vi "Teleop.vi"(10 "Match Info":T1={"Autonomous Elapsed Seconds"=0.0, "TeleOp Elapsed Seconds"=0.0, "Disabled Elapsed Seconds"=0.0, "Visited Autonomous"=FALSE, "Visited TeleOp"=FALSE, "Visited Disabled"=FALSE, "Autonomous Settings"={"Autonomous Style"=enum."Independent", "VI Refnum"=refnum}}, 11 "Call Context":T2) -> ()   [LabVIEW 2018]
doc: "This VI is called for each enabled TeleOp packet received from the DS. It is typically used to read from joysticks and other inputs and update I/O or setpoints for timed control loops. It should complete and return within 20 milliseconds or risk missing DS packets."
uses:
  <vilib>/Rock Robotics/WPI/DriverStation/WPI_DriverStationDerivedRobotMode.ctl
  <vilib>/Rock Robotics/WPI/DriverStation/WPI_DriverStationMatch Info.ctl
  <vilib>/Rock Robotics/WPI/Solenoid/WPI_SolenoidValue.ctl
  Framework/Robot Global Data.vi
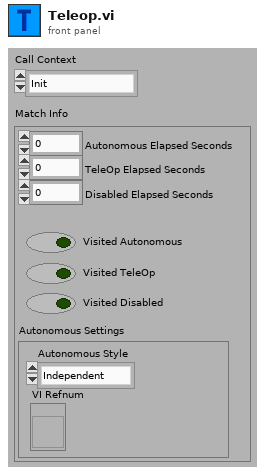
[diagram p1: front panel]
types:
  T1 = typedef "WPI_DriverStationMatch Info.ctl" = cluster{"Autonomous Elapsed Seconds":dbl, "TeleOp Elapsed Seconds":dbl, "Disabled Elapsed Seconds":dbl, "Visited Autonomous":bool, "Visited TeleOp":bool, "Visited Disabled":bool, "Autonomous Settings":cluster{"Autonomous Style":enum16{"Iterative", "Independent"}, "VI Refnum":refnum<vi>}}
  T2 = typedef "WPI_DriverStationDerivedRobotMode.ctl" = enum16{"Init", "Execute", "Stop"}
  T3 = typedef "Command Status Info.ctl" = cluster{"Name":string, "Status":T4, "notifier out":T5}
  T4 = typedef "Completion Status.ctl" = enum16{"Successful", "Aborted", "Incomplete"}
  T5 = typedef "Completion Notifier.ctl" = refnum<notifier>
  T6 = typedef "WPI_SolenoidValue.ctl" = enum16{"Off", "On", "Forward", "Reverse"}
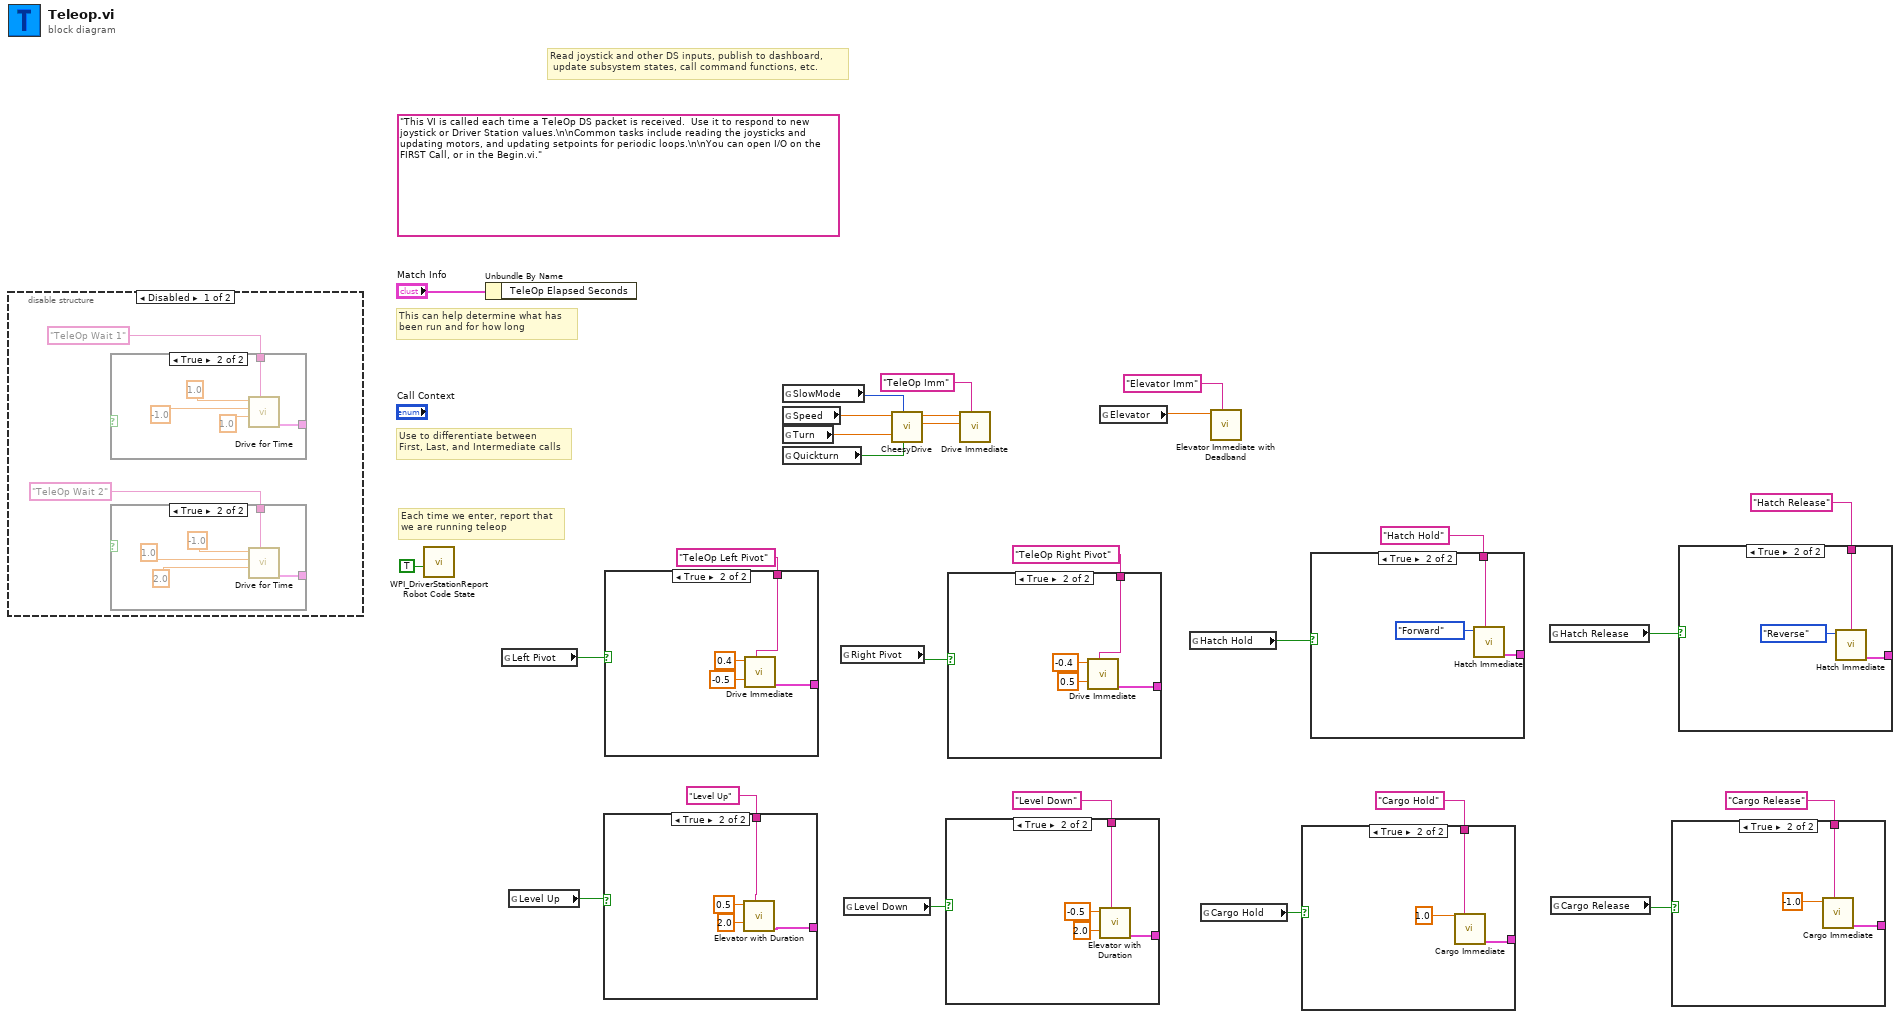
[diagram p0: block diagram]
diagram:
  (unwired) "This VI is called each time a TeleOp DS packet is received.  Use it to respond to new joystick or Driver Station values.\n\nCommon tasks include reading the joysticks and updating motors, and updating setpoints for periodic loops.\n\nYou can open I/O on the FIRST Call, or in the Begin.vi."
  # "Read joystick and other DS inputs, publish to dashboard,\n update subsystem states, call command functions, etc."
  # "Each time we enter, report that\nwe are running teleop"
  # "Use to differentiate between\nFirst, Last, and Intermediate calls"
  # "This can help determine what has\nbeen run and for how long"
  n1 = disable-structure shown="Disabled" {
    frame Disabled {
      n2 = case shown="True" w29 {
        tunnel: [_ w40] -> _
        tunnel: "TeleOp Wait 1" ("Description") -> [_ w39]
        frame False {
        }
        frame True {
          n3 = call "Drive for Time.vi"("Description"=w39, "Seconds"=1.0, "Right Speed"=-1.0, "Left Speed"=1.0) -> ("Command Info Out"=w40:T3)  [unwired: 7 in]
        }
      }
      n4 = case shown="True" w28 {
        tunnel: [_ w34] -> _
        tunnel: "TeleOp Wait 2" ("Description") -> [_ w33]
        frame False {
        }
        frame True {
          n5 = call "Drive for Time.vi"("Description"=w33, "Seconds"=2.0, "Right Speed"=1.0, "Left Speed"=-1.0) -> ("Command Info Out"=w34:T3)  [unwired: 7 in]
        }
      }
    }
    frame Enabled {
    }
  }
  n6 = call <vilib>:"WPI_DriverStationReport Robot Code State.vi"("TeleOp"=TRUE ("Autonomous")) -> ()  [unwired: 10 in, 1 out]
  n7 = Unbundle By Name("Match Info") -> ()  [unwired: 1 out]
  n8 = global read "Robot Global Data.vi" "Left Pivot"() -> (w16:bool)
  n9 = global read "Robot Global Data.vi" "Level Up"() -> (w12:bool)
  n10 = case shown="True" w12 {
    tunnel: [_ w45] -> _
    tunnel: "Level Up" ("Description") -> [_ w44]
    frame False {
    }
    frame True {
      n11 = call "Elevator with Duration.vi"("Description"=w44, "Duration (s)"=2.0, "Setpoint"=0.5) -> ("Command Info Out"=w45:T3)  [unwired: 8 in]
    }
  }
  n12 = case shown="True" w16 {
    tunnel: [_ w47] -> _
    tunnel: "TeleOp Left Pivot" ("Description") -> [_ w46]
    frame False {
    }
    frame True {
      n13 = call "Drive Immediate.vi"("Description"=w46, "Right Setpoint"=-0.5, "Left Setpoint"=0.4) -> ("Command Info Out"=w47:T3)  [unwired: 8 in]
    }
  }
  n14 = global read "Robot Global Data.vi" "SlowMode"() -> (w15:u32)
  n15 = global read "Robot Global Data.vi" "Speed"() -> (w22:dbl)
  n16 = global read "Robot Global Data.vi" "Turn"() -> (w21:dbl)
  n17 = global read "Robot Global Data.vi" "Quickturn"() -> (w20:bool)
  n18 = global read "Robot Global Data.vi" "Right Pivot"() -> (w17:bool)
  n19 = global read "Robot Global Data.vi" "Level Down"() -> (w11:bool)
  n20 = call "CheesyDrive.vi"("Quickturn"=w20, "SlowMode"=w15, "Wheel"=w21, "Throttle"=w22) -> ("Right PWM"=w23:dbl, "Left PWM"=w24:dbl)  [unwired: 6 in]
  n21 = case shown="True" w11 {
    tunnel: "Level Down" ("Description") -> [_ w53]
    tunnel: [_ w52] -> _
    frame False {
    }
    frame True {
      n22 = call "Elevator with Duration.vi"("Description"=w53, "Duration (s)"=2.0, "Setpoint"=-0.5) -> ("Command Info Out"=w52:T3)  [unwired: 8 in]
    }
  }
  n23 = case shown="True" w17 {
    tunnel: [_ w55] -> _
    tunnel: "TeleOp Right Pivot" ("Description") -> [_ w54]
    frame False {
    }
    frame True {
      n24 = call "Drive Immediate.vi"("Description"=w54, "Right Setpoint"=0.5, "Left Setpoint"=-0.4) -> ("Command Info Out"=w55:T3)  [unwired: 8 in]
    }
  }
  n25 = call "Drive Immediate.vi"("Description"="TeleOp Imm", "Right Setpoint"=w23, "Left Setpoint"=w24) -> ()  [unwired: 8 in, 1 out]
  n26 = global read "Robot Global Data.vi" "Elevator"() -> (w6:dbl)
  n27 = global read "Robot Global Data.vi" "Hatch Hold"() -> (w1:bool)
  n28 = global read "Robot Global Data.vi" "Cargo Hold"() -> (w8:bool)
  n29 = call "Elevator Immediate with Deadband.vi"("Description"="Elevator Imm", "Setpoint"=w6) -> ()  [unwired: 9 in, 1 out]
  n30 = case shown="True" w8 {
    tunnel: [_ w60] -> _
    tunnel: "Cargo Hold" ("Description") -> [_ w59]
    frame False {
    }
    frame True {
      n31 = call "Cargo Immediate.vi"("Description"=w59, "Setpoint"=1.0 ("Left Setpoint")) -> ("Command Info Out"=w60:T3)  [unwired: 9 in]
    }
  }
  n32 = case shown="True" w1 {
    tunnel: "Hatch Hold" ("Description") -> [_ w63]
    tunnel: [_ w62] -> _
    frame False {
    }
    frame True {
      n33 = call "Hatch Immediate.vi"("Description"=w63, "Hatch Action"=WPI_SolenoidValue."Forward") -> ("Command Info Out"=w62:T3)  [unwired: 9 in]
    }
  }
  n34 = global read "Robot Global Data.vi" "Hatch Release"() -> (w2:bool)
  n35 = global read "Robot Global Data.vi" "Cargo Release"() -> (w7:bool)
  n36 = case shown="True" w7 {
    tunnel: [_ w66] -> _
    tunnel: "Cargo Release" ("Description") -> [_ w64]
    frame False {
    }
    frame True {
      n37 = call "Cargo Immediate.vi"("Description"=w64, "Setpoint"=-1.0 ("Left Setpoint")) -> ("Command Info Out"=w66:T3)  [unwired: 9 in]
    }
  }
  n38 = case shown="True" w2 {
    tunnel: "Hatch Release" ("Description") -> [_ w69]
    tunnel: [_ w68] -> _
    frame False {
    }
    frame True {
      n39 = call "Hatch Immediate.vi"("Description"=w69, "Hatch Action"=WPI_SolenoidValue."Reverse") -> ("Command Info Out"=w68:T3)  [unwired: 9 in]
    }
  }
